vi "Clear.vi"(8 "error in (no error)":errorcluster, 11 "ResultTree in":refnum<class "ResultTree.lvclass">) -> (0 "error out":errorcluster, 3 "ResultTree out":refnum<class "ResultTree.lvclass">)   [LabVIEW 2017, in "ResultTree.lvclass"]
doc: "Removes all items from the tree."
uses:
  ResultTree.lvclass
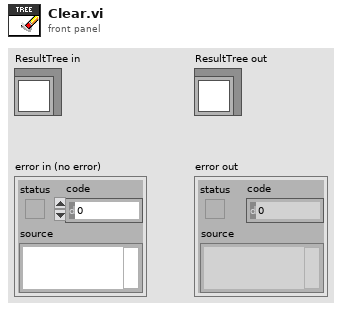
[diagram p1: front panel]
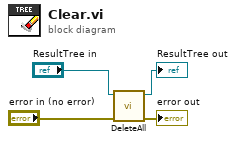
[diagram p0: block diagram]
diagram:
  n1 = call "DeleteAll.vi"("error in (no error)"="error in (no error)", "ResultTree in"="ResultTree in") -> ("error out"=→"error out":errorcluster, "ResultTree out"=→"ResultTree out":refnum<class "ResultTree.lvclass">)  [unwired: 8 in]
